vi "FdT.vi"() -> ()   [LabVIEW 2022 SP3]
uses:
  <vilib>/Instr/_visa.llb/VISA Configure Serial Port (Instr).vi
panel:
  out "Numeric":dbl
  in  "VISA resource name":refnum<visa-resource-name>
  in  "Stop Button":bool
  out "Waveform Chart":cluster{i32}(graph)
  in  "Velocidad":dbl
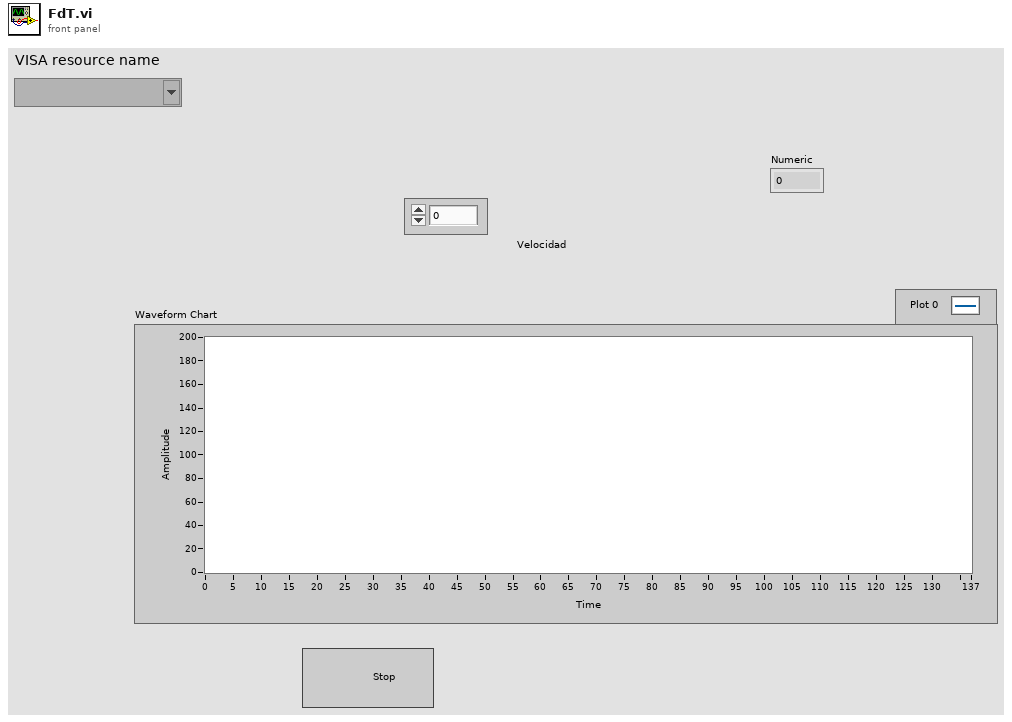
[diagram p1: front panel]
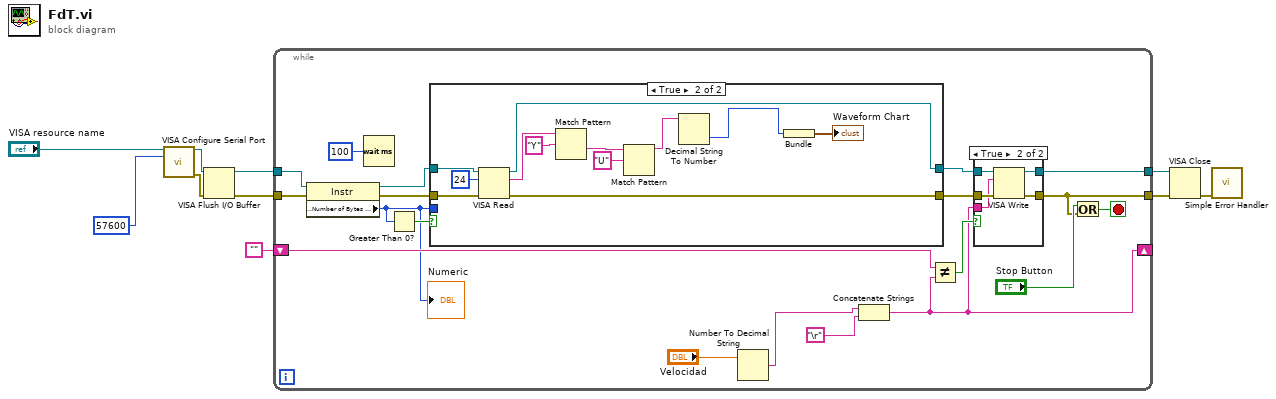
[diagram p0: block diagram]
diagram:
  n1 = call-poly "VISA Configure Serial Port"("VISA resource name"="VISA resource name", "baud rate (9600)"=u32 57600) -> ("VISA resource name out"=w4:refnum<visa-resource-name>, "error out"=w3:errorcluster)  [unwired: 12 in]
  n2 = VISA Flush I/O Buffer(VISA resource name=w4, error in (no error)=w3) -> (VISA resource name out=w2:refnum<visa-resource-name>, error out=w1:errorcluster)  [unwired: 1 in]
  n3 = while {
    tunnel: [w29] -> w10
    tunnel: [w22] -> w9
    shift-right: [w25] -> _
    shift-left: "" -> [w26]
    tunnel: w2 -> [w21]
    tunnel: w1 -> [w20]
    stop <- w28 stop-if-true
    n4 = property class="Instr"(reference=w21, error in=w20) -> (reference out=w19:refnum<visa-resource-name>, error out=w18:errorcluster, "Serial Settings:Number of Bytes at Serial Port"=w12:u32)
    "Numeric" <- w12
    n5 = Wait (ms)(milliseconds to wait=u32 100) -> ()  [unwired: 1 out]
    n6 = Greater Than 0?(x=w12) -> (x > 0?=w15:bool)
    n7 = case shown="True" w15 {
      tunnel: w19 -> [w31 w43]
      tunnel: w18 -> [w30 w42]
      tunnel: [w31 w41] -> w17
      tunnel: [w30 w40] -> w16
      tunnel: w12 -> [_ _]
      frame False {
      }
      frame True {
        n8 = VISA Read(VISA resource name=w43, byte count=u32 24, error in (no error)=w42) -> (VISA resource name out=w41:refnum<visa-resource-name>, read buffer=w38:string, error out=w40:errorcluster)  [unwired: 1 out]
        n9 = Match Pattern(string=w38, regular expression="Y") -> (after substring=w34:string)  [unwired: 1 in, 3 out]
        n10 = Match Pattern(string=w34, regular expression="U") -> (before substring=w33:string)  [unwired: 1 in, 3 out]
        n11 = Decimal String To Number(string=w33) -> (number=w36:i32)  [unwired: 2 in, 1 out]
        n12 = Bundle(w36) -> (→"Waveform Chart":cluster{i32})  [unwired: 1 in]
      }
    }
    n13 = Number To Decimal String(number="Velocidad") -> (decimal integer string=w11:string)  [unwired: 1 in]
    n14 = Concatenate Strings(w11, "\r") -> (w25:string)
    n15 = Not Equal?(x=w26, y=w25) -> (x != y?=w27:bool)
    n16 = case shown="True" w27 {
      tunnel: w17 -> [w45 w50]
      tunnel: [w45 w49] -> w29
      tunnel: w16 -> [w44 w48]
      tunnel: [w44 w47] -> w22
      tunnel: w25 -> [_ w46]
      frame False {
      }
      frame True {
        n17 = VISA Write(VISA resource name=w50, write buffer=w46, error in (no error)=w48) -> (VISA resource name out=w49:refnum<visa-resource-name>, error out=w47:errorcluster)  [unwired: 1 out]
      }
    }
    n18 = Or(x="Stop Button", y=w22) -> (x .or. y?=w28:bool)
  }
  n19 = VISA Close(VISA resource name=w10, error in (no error)=w9) -> (error out=w7:errorcluster)
  n20 = call <vilib>:"Simple Error Handler.vi"("error in (no error)"=w7) -> ()  [unwired: 4 in, 5 out]
